vi "Image Path Dialog.vi"(8 "error in (no error)":errorcluster, 10 "Default Name":string, 11 "Start Path (Default: Last)":path=path "") -> (0 "error out":errorcluster, 1 "Cancelled?":bool, 2 "Saved Image File Format":T1, 3 "Selected Path":path, 4 "Exists?":bool caption="exists")   [LabVIEW 2019]
uses:
  Pictures/Save File Format.ctl
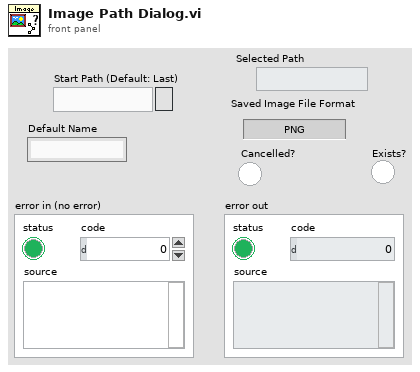
[diagram p1: front panel]
types:
  T1 = typedef "Save File Format.ctl" = enum16{"PNG", "JPEG", "BMP"}
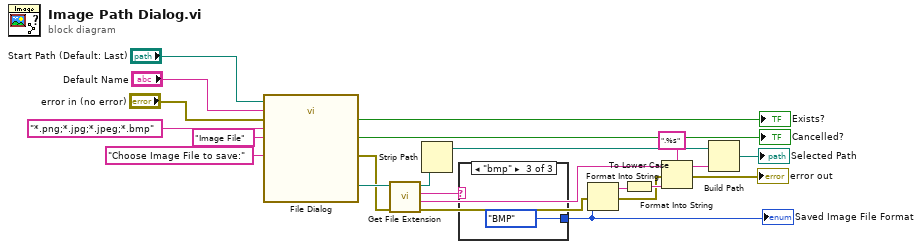
[diagram p0: block diagram]
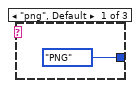
[diagram p2: hidden frame]
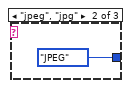
[diagram p3: hidden frame]
diagram:
  n1 = call "File Dialog"("start path"="Start Path (Default: Last)", "prompt"="Choose Image File to save:", "default name"="Default Name", "error in"="error in (no error)", "pattern (all files)"="*.png;*.jpg;*.jpeg;*.bmp", "pattern label"="Image File") -> ("selected path"=w20:path, "exists"=→"Exists?":bool, "cancelled"=→"Cancelled?":bool, "error out"=w19:errorcluster)  [unwired: 6 in]
  n2 = call <vilib>:"Get File Extension.vi"("error in (no error)"=w19, "file"=w20) -> ("error out"=w11:errorcluster, "filename without extension"=w9:string, "lowercase file extension"=w18:string, "dup file"=w6:path)  [unwired: 5 in, 1 out]
  n3 = Strip Path(path=w6) -> (stripped path=w4:path)  [unwired: 1 out]
  n4 = case shown="\"bmp\"" w18 {
    tunnel: [Save_File_Format."PNG" ("Saved Image File Format") Save_File_Format."JPEG" ("Saved Image File Format") Save_File_Format."BMP" ("Saved Image File Format")] -> w13
    frame "png", Default {
    }
    frame "jpeg", "jpg" {
    }
    frame "bmp" {
    }
  }
  "Saved Image File Format" <- w13
  n5 = Format Into String(error in=w11, w13) -> (resulting string=w12:string, error out=w8:errorcluster)  [unwired: 2 in]
  n6 = To Lower Case(string=w12) -> (all lower case string=w10:string)
  n7 = Format Into String(format string=".%s", initial string=w9, error in=w8, w10) -> (resulting string=w5:string, error out=→"error out":errorcluster)
  n8 = Build Path(base path=w4, name or relative path=w5) -> (appended path=→"Selected Path":path)
